vi "Add actual date time to string.vi"(4 "String in":string) -> (1 "String out":string)   [LabVIEW 2021, in "MatS Libs.lvlib"]
doc: "Adds current date and time (yyyy-mm-dd HH.MM.SS) in front of the string. Underscore is used to separate date+time from the string.\nUsefull for logging of messages or creating filenames."
uses:
  <userlib>/MatS Libs/MatS Libs.lvlib
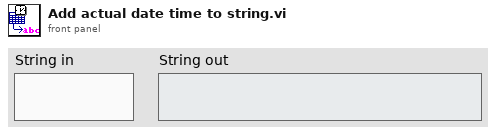
[diagram p1: front panel]
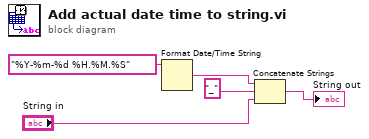
[diagram p0: block diagram]
diagram:
  n1 = Format Date/Time String(time format string (%c)="%Y-%m-%d %H.%M.%S") -> (date/time string=w2:string)  [unwired: 2 in]
  n2 = Concatenate Strings(w2, "_" ("string"), "String in") -> (→"String out":string)
